vi "Subvi counter up U16.vi"(4 "Reset":bool, 9 "+1":bool) -> (1 "Output":u16)   [LabVIEW 2017]
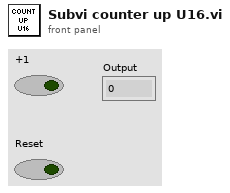
[diagram p1: front panel]
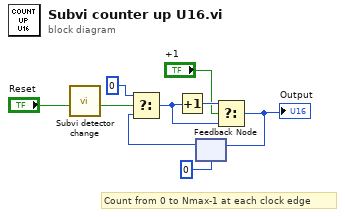
[diagram p0: block diagram]
diagram:
  # "Count from 0 to Nmax-1 at each clock edge"
  n1 = call "Subvi detector change.vi"("Input"="Reset") -> ("Output"=w3:bool)  [unwired: 8 in]
  n2 = feedback #1(u16 0) -> (w5:u16)
  n3 = Select(t=u16 0, s=w3, f=w5) -> (s? t:f=w6:u16)
  n4 = Increment(x=w6) -> (x+1=w7:u16)
  n5 = Select(t=w7, s="+1", f=w6) -> (s? t:f=w8:u16)
  "Output" <- w8
  n6 = feedback-in #1(w8) -> ()
